vi "Static Block Lock.vi"(9 "Block Option":T1, 11 "PN532 COM Port":refnum<visa-resource-name>) -> (0 "Error out":errorcluster, 2 "Succeeded":bool, 3 "PN532 COM Port Out":refnum<visa-resource-name>)   [LabVIEW 2012, in "NFC Driver.lvlib"]
uses:
  NFC Driver.lvlib
  Typedef/Static Block Lock Section.ctl
panel:
  out "result string":string
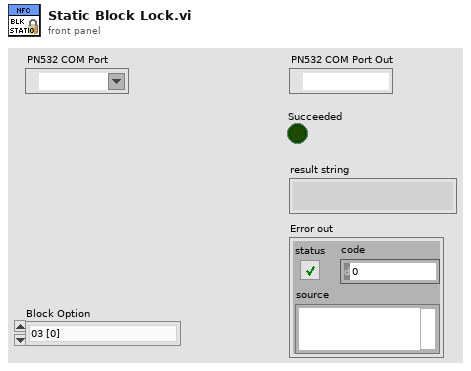
[diagram p1: front panel]
types:
  T1 = typedef "NFC Driver.lvlib/Static Block Lock Section.ctl" = enum16{"03 [0]", "04-09 [1]", "10-15 [2]"}
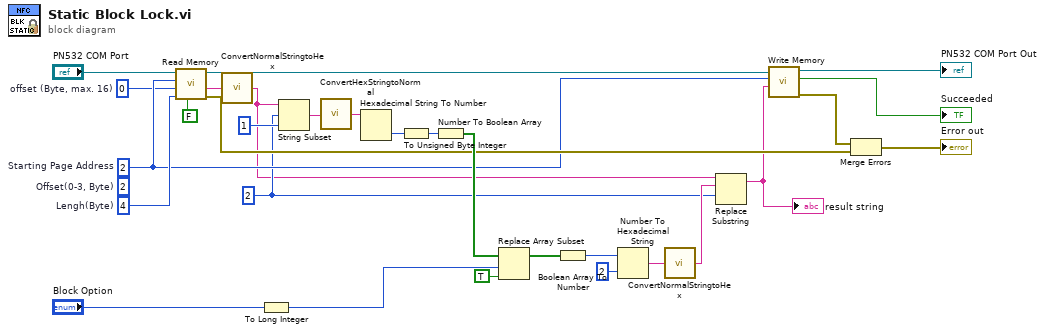
[diagram p0: block diagram]
diagram:
  w10 = 2
  w13 = 0  # offset (Byte, max. 16)
  (unwired) 2  # Offset(0-3, Byte)
  w27 = 4  # Lengh(Byte)
  w17 = 2  # Starting Page Address
  n1 = call "Read Memory.vi"("Reverse Output[F]"=FALSE, "length (Byte, max. 16)"=w27, "offset (Byte, max. 16)"=w13, "Page Address"=w17, "PN532 COM Port"="PN532 COM Port") -> ("error out"=w21:errorcluster, "Selected substring (HEX)"=w3:string, "PN532 COM Port Out"=w1:refnum<visa-resource-name>)  [unwired: 2 in, 2 out]
  n2 = call "ConvertNormalStringtoHex.vi"("Normal String"=w3) -> ("Hex String"=w9:string)
  n3 = To Long Integer(number="Block Option") -> (32bit integer=w6:i32)
  n4 = String Subset(string=w9, offset (0)=w10, length (rest)=1 ("length (rest)")) -> (substring=w15:string)
  n5 = call "ConvertHexStringtoNormal.vi"("Hex String"=w15) -> ("Normal String"=w14:string)
  n6 = Hexadecimal String To Number(string=w14) -> (number=w26:u32)  [unwired: 2 in, 1 out]
  n7 = To Unsigned Byte Integer(number=w26) -> (unsigned 8bit integer=w18:u8)
  n8 = Number To Boolean Array(number=w18) -> (Boolean array=w25:bool[])
  n9 = Replace Array Subset(array=w25, new element=TRUE ("new element/subarray"), index=w6) -> (w20:bool[])
  n10 = Boolean Array To Number(Boolean array=w20) -> (number=w24:u32)
  n11 = Number To Hexadecimal String(1:i16 2 ("width (-)"), 2:w24) -> (0:w12:string)
  n12 = call "ConvertNormalStringtoHex.vi"("Normal String"=w12) -> ("Hex String"=w11:string)
  n13 = Replace Substring(3:w10, 4:w11, 5:w9) -> (1:w8:string)  [unwired: 1 in, 1 out]
  "result string" <- w8
  n14 = call "Write Memory.vi"("Data to write (HEX, max 16 bytes)"=w8, "Page Address"=w17, "PN532 COM Port"=w1) -> ("Error Out"=w22:errorcluster, "Succesful?"=→"Succeeded":bool, "PN532 COM Port Out"=→"PN532 COM Port Out":refnum<visa-resource-name>)  [unwired: 6 in]
  n15 = Merge Errors(w22, w21) -> (→"Error out":errorcluster)
